vi "String Trigger independiente (SubVI).vi"(2 "Holdoff":dbl(knob) scale=5e-07..10.0, 3 "Nivel":dbl(knob) scale=-20.0..20.0, 4 "Mode":u16(ring) items=["Auto", "Normal"], 5 "Force":bool, 6 "State":bool, 7 "Frecuency":bool) -> (1 "String trigges independiente":string)   [LabVIEW 2019]
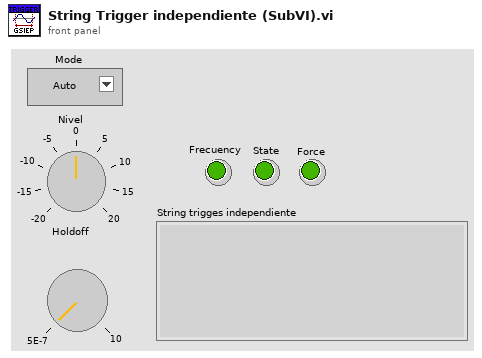
[diagram p1: front panel]
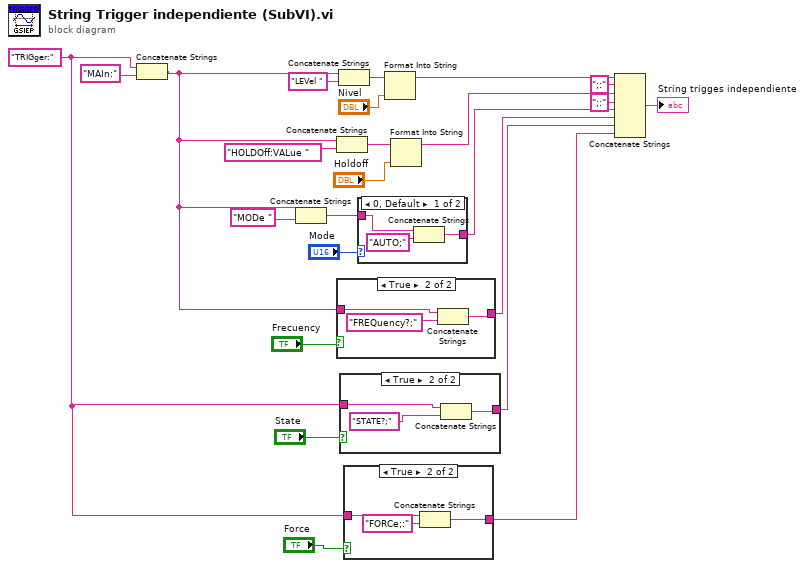
[diagram p0: block diagram]
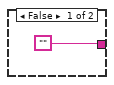
[diagram p2: hidden frame]
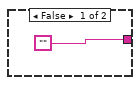
[diagram p3: hidden frame]
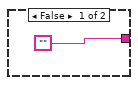
[diagram p4: hidden frame]
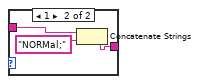
[diagram p5: hidden frame]
diagram:
  w3 = "TRIGger:"
  n1 = Concatenate Strings(w3, "MAIn:") -> (w7:string)
  n2 = Concatenate Strings(w7, "MODe ") -> (w16:string)
  n3 = Concatenate Strings(w7, "HOLDOff:VALue ") -> (w20:string)
  n4 = case shown="True" "Frecuency" {
    tunnel: w7 -> [_ w27]
    tunnel: ["" w26] -> w9
    frame False {
    }
    frame True {
      n5 = Concatenate Strings(w27, "FREQuency?;") -> (w26:string)
    }
  }
  n6 = Concatenate Strings(w7, "LEVel ") -> (w23:string)
  n7 = case shown="True" "State" {
    tunnel: w3 -> [_ w32]
    tunnel: ["" w30] -> w5
    frame False {
    }
    frame True {
      n8 = Concatenate Strings(w32, "STATE?;") -> (w30:string)
    }
  }
  n9 = case shown="True" "Force" {
    tunnel: w3 -> [_ w35]
    tunnel: ["" w34] -> w2
    frame False {
    }
    frame True {
      n10 = Concatenate Strings(w35, "FORCe;:") -> (w34:string)
    }
  }
  n11 = case shown="0, Default" "Mode" {
    tunnel: w16 -> [w39 w42]
    tunnel: [w37 w40] -> w10
    frame 0, Default {
      n12 = Concatenate Strings(w39, "AUTO;") -> (w37:string)
    }
    frame 1 {
      n13 = Concatenate Strings(w42, "NORMal;") -> (w40:string)
    }
  }
  n14 = Format Into String(initial string=w23, "Nivel") -> (resulting string=w14:string)  [unwired: 2 in, 1 out]
  n15 = Format Into String(initial string=w20, "Holdoff") -> (resulting string=w12:string)  [unwired: 2 in, 1 out]
  n16 = Concatenate Strings(w14, ";:", w12, ";:", w10, w9, w5, w2) -> (→"String trigges independiente":string)
